vi "CCP_tcp_server.vi"(5 "timeout":i32=1000, 6 "value":refnum<vi>, 7 "port":u16=9999, 8 "error_in":errorcluster, 11 "conn_id_in":refnum<k5>) -> (0 "error_out":errorcluster, 3 "conn_id_out":refnum<k5>, 4 "status":string)   [LabVIEW 2019]
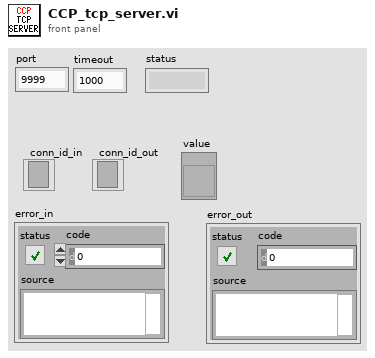
[diagram p1: front panel]
types:
  T1 = enum16{"Standard", "Buffered", "CRLF", "Immediate"}
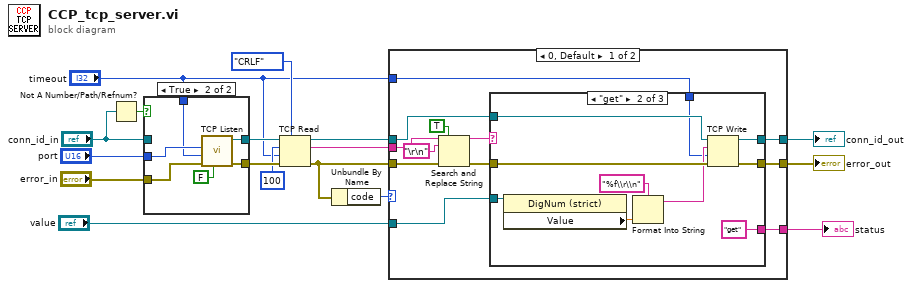
[diagram p0: block diagram]
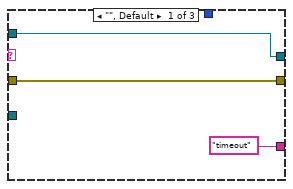
[diagram p2: hidden frame]
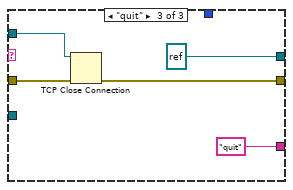
[diagram p3: hidden frame]
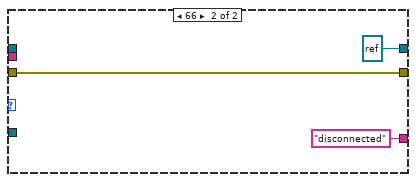
[diagram p4: hidden frame]
diagram:
  n1 = Not A Number/Path/Refnum?(number/path/refnum="conn_id_in") -> (NaN/Path/Refnum?=w17:bool)
  n2 = case shown="True" w17 {
    tunnel: [w19 w25] -> w14
    tunnel: "conn_id_in" -> [w19 _]
    tunnel: "port" -> [_ w24]
    tunnel: "timeout" -> [_ w23]
    tunnel: [w18 w21] -> w12
    tunnel: "error_in" -> [w18 w20]
    frame False {
    }
    frame True {
      n3 = call <vilib>:"TCP Listen.vi"("resolve remote address (T)"=FALSE, "error in (no error)"=w20, "timeout ms (wait forever: -1)"=w23, "port"=w24) -> ("error out"=w21:errorcluster, "connection ID"=w25:refnum<k5>)  [unwired: 3 in, 3 out]
    }
  }
  n4 = TCP Read(connection ID=w14, bytes to read=100, error in (no error)=w12, 7:T1."CRLF" ("mode (standard)"), 9:"timeout") -> (connection ID out=w8:refnum<k5>, data out=w9:string, error out=w2:errorcluster)
  n5 = Unbundle By Name(w2) -> ("code"=w1:i32)
  n6 = case shown="0, Default" w1 {
    tunnel: w9 -> [w37 _]
    tunnel: w8 -> [w33 _]
    tunnel: [w31 w57] -> w7
    tunnel: "value" -> [w30 _]
    tunnel: "timeout" -> [w29 _]
    tunnel: [w28 refnum<k5> refnum ("conn_id 2")] -> w4
    tunnel: [w27 "disconnected"] -> w3
    tunnel: w2 -> [w26 w57]
    frame 0, Default {
      n7 = Search and Replace String(replace all?=TRUE ("replace all? (F)"), input string=w37, search string="\r\n", error in=w26) -> (result string=w34:string, error out=w32:errorcluster)  [unwired: 4 in, 2 out]
      n8 = case shown="\"get\"" w34 {
        tunnel: w33 -> [w40 w44 w55]
        tunnel: w32 -> [w39 w48 w54]
        tunnel: [w40 w43 refnum<k5> refnum ("conn_id 2")] -> w28
        tunnel: [w39 w49 w52] -> w31
        tunnel: w30 -> [_ w50 _]
        tunnel: w29 -> [_ w42 _]
        tunnel: ["timeout" "get" "quit"] -> w27
        frame "", Default {
        }
        frame "get" {
          n9 = property on="Property Node" class="DigNum (strict)"(reference=w50) -> ("Value"=w46:dbl)  [unwired: 1 in, 2 out]
          n10 = Format Into String(format string="%f\\r\\n", w46) -> (resulting string=w45:string)  [unwired: 2 in, 1 out]
          n11 = TCP Write(connection ID=w44, data in=w45, error in (no error)=w48, 9:w42) -> (connection ID out=w43:refnum<k5>, error out=w49:errorcluster)  [unwired: 1 out]
        }
        frame "quit" {
          n12 = TCP Close Connection(connection ID=w55, error in (no error)=w54) -> (error out=w52:errorcluster)  [unwired: 1 in, 1 out]
        }
      }
    }
    frame 66 {
    }
  }
  "status" <- w3
  "error_out" <- w7
  "conn_id_out" <- w4
